vi "Boolean Output Item UI Update.vi"(8 "error in (no error)":errorcluster, 10 "Bool UI Elements":T1, 11 "Output":T2) -> (0 "error out":errorcluster)   [LabVIEW 2015, in "OutputUI.lvclass"]
uses:
  OutputUI.lvclass
  Step/STEP_OUTPUT.ctl
  Step/OUTPUT_DATA_TYPE.ctl
  OUTPUT_CHECK_TYPE.ctl
  Step/OUTPUT_VALUE_TYPE.ctl
  Step.lvclass
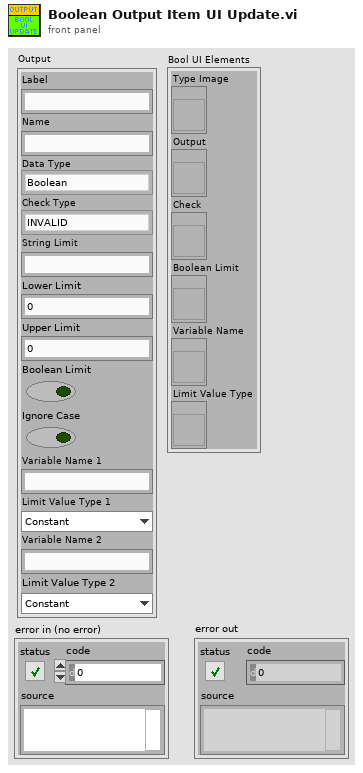
[diagram p1: front panel]
types:
  T1 = cluster{"Type Image":refnum<vi>, "Output":refnum<vi>, "Check":refnum<vi>, "Boolean Limit":refnum<vi>, "Variable Name":refnum<vi>, "Limit Value Type":refnum<vi>}
  T2 = typedef "Step.lvclass/STEP_OUTPUT.ctl" = cluster{"Label":string, "Name":string, "Data Type":T3, "Check Type":T4, "String Limit":string, "Lower Limit":dbl, "Upper Limit":dbl, "Boolean Limit":bool, "Ignore Case":bool, "Variable Name 1":string, "Limit Value Type 1":T5, "Variable Name 2":string, "Limit Value Type 2":T5}
  T3 = typedef "Step.lvclass/OUTPUT_DATA_TYPE.ctl" = enum16{"Boolean", "String", "Numeric", "Other"}
  T4 = typedef "Step.lvclass/OUTPUT_CHECK_TYPE.ctl" = enum16{"INVALID", "DO_NOT_CHECK", "RECORD", "VARIABLE", "EQUAL", "NOT_EQUAL", "STR_CONTAINS", "STR_START_WITH", "STR_END_WITH", "STR_REGEX_MATCH", "NUM_GT", "NUM_LT", "NUM_GE", "NUM_LE", "NUM_RANGE", "NUM_RANGE_BDY"}
  T5 = typedef "Step.lvclass/OUTPUT_VALUE_TYPE.ctl" = enum16{"Constant", "Variable"}
  T6 = enum8{"Enabled", "Disabled", "Disabled and Grayed Out"}
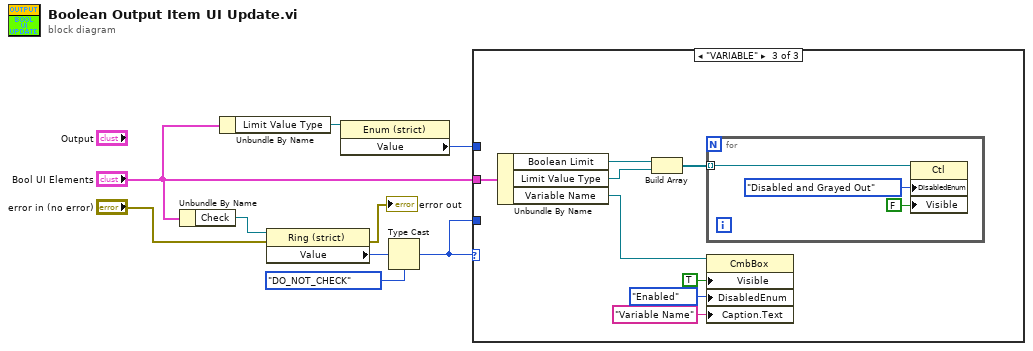
[diagram p0: block diagram]
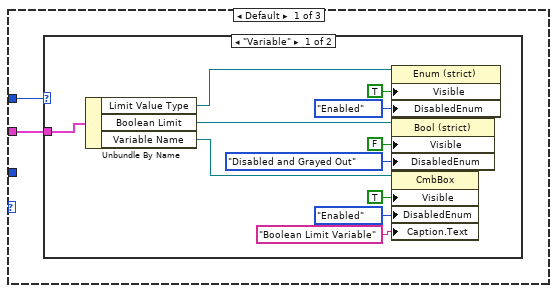
[diagram p2: hidden frame]
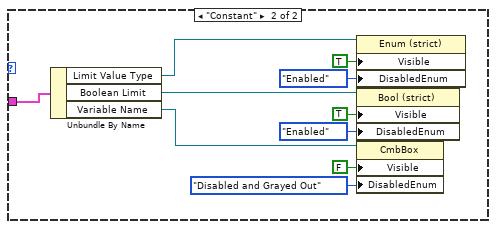
[diagram p3: hidden frame]
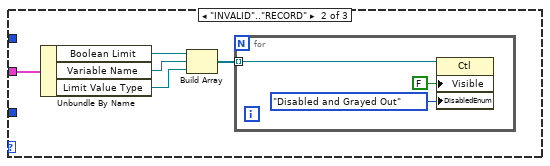
[diagram p4: hidden frame]
diagram:
  n1 = Unbundle By Name("Bool UI Elements") -> ("Check"=w9:refnum<vi>)
  n2 = Unbundle By Name("Bool UI Elements") -> ("Limit Value Type"=w2:refnum<vi>)
  n3 = property class="Ring (strict)"(reference=w9, error in="error in (no error)") -> (error out=→"error out":errorcluster, "Value"=w7:u16)  [unwired: 1 out]
  n4 = property class="Enum (strict)"(reference=w2) -> ("Value"=w1:T5)  [unwired: 1 in, 2 out]
  n5 = Type Cast(type=OUTPUT_CHECK_TYPE."DO_NOT_CHECK" ("Check Type"), x=w7) -> (*(type *) &x=w6:T4)
  n6 = case shown="\"VARIABLE\"" w6 {
    tunnel: w6 -> [_ _ _]
    tunnel: "Bool UI Elements" -> [w11 w33 w48]
    tunnel: w1 -> [w10 _ _]
    frame Default {
      n7 = case shown="\"Variable\"" w10 {
        tunnel: w11 -> [w22 w32]
        frame "Variable" {
          n8 = Unbundle By Name(w22) -> ("Limit Value Type"=w17:refnum<vi>, "Boolean Limit"=w20:refnum<vi>, "Variable Name"=w21:refnum<vi>)
          n9 = property class="Enum (strict)"(reference=w17, "Visible"=TRUE, "DisabledEnum"=T6."Enabled" ("Disabled")) -> ()  [unwired: 1 in, 2 out]
          n10 = property class="Bool (strict)"(reference=w20, "Visible"=FALSE, "DisabledEnum"=T6."Disabled and Grayed Out" ("Disabled")) -> ()  [unwired: 1 in, 2 out]
          n11 = property class="CmbBox"(reference=w21, "Visible"=TRUE, "DisabledEnum"=T6."Enabled" ("Disabled"), "Caption.Text"="Boolean Limit Variable" ("format string")) -> ()  [unwired: 1 in, 2 out]
        }
        frame "Constant" {
          n12 = Unbundle By Name(w32) -> ("Limit Value Type"=w27:refnum<vi>, "Boolean Limit"=w30:refnum<vi>, "Variable Name"=w31:refnum<vi>)
          n13 = property class="Enum (strict)"(reference=w27, "Visible"=TRUE, "DisabledEnum"=T6."Enabled" ("Disabled")) -> ()  [unwired: 1 in, 2 out]
          n14 = property class="Bool (strict)"(reference=w30, "Visible"=TRUE, "DisabledEnum"=T6."Enabled" ("Disabled")) -> ()  [unwired: 1 in, 2 out]
          n15 = property class="CmbBox"(reference=w31, "Visible"=FALSE, "DisabledEnum"=T6."Disabled and Grayed Out" ("Disabled")) -> ()  [unwired: 1 in, 2 out]
        }
      }
    }
    frame "INVALID".."RECORD" {
      n16 = Unbundle By Name(w33) -> ("Boolean Limit"=w37:refnum<vi>, "Variable Name"=w36:refnum<vi>, "Limit Value Type"=w35:refnum<vi>)
      n17 = Build Array(w37, w36, w35) -> (w34:refnum<vi>[])
      n18 = for {
        tunnel: w34 -> [w40] mode=indexing
        n19 = property class="Ctl"(reference=w40, "Visible"=FALSE, "DisabledEnum"=T6."Disabled and Grayed Out" ("Disabled")) -> ()  [unwired: 1 in, 2 out]
      }
    }
    frame "VARIABLE" {
      n20 = Unbundle By Name(w48) -> ("Boolean Limit"=w47:refnum<vi>, "Limit Value Type"=w46:refnum<vi>, "Variable Name"=w42:refnum<vi>)
      n21 = Build Array(w47, w46) -> (w45:refnum<vi>[])
      n22 = for {
        tunnel: w45 -> [w51] mode=indexing
        n23 = property class="Ctl"(reference=w51, "DisabledEnum"=T6."Disabled and Grayed Out" ("Disabled"), "Visible"=FALSE) -> ()  [unwired: 1 in, 2 out]
      }
      n24 = property class="CmbBox"(reference=w42, "Visible"=TRUE, "DisabledEnum"=T6."Enabled" ("Disabled"), "Caption.Text"="Variable Name" ("format string")) -> ()  [unwired: 1 in, 2 out]
    }
  }
